vi "read_inverter (SubVI).vi"(8 "error in (no error)":errorcluster, 11 "Modbus Master in":refnum<class "Modbus Master.lvclass">) -> (0 "error out":errorcluster, 3 "Modbus Master out":refnum<class "Modbus Master.lvclass">)   [LabVIEW 2024, in "SALICRU_MODBUS.lvlib"]
uses:
  SALICRU_MODBUS.lvlib
  <vilib>/Modbus/master/Modbus Master.lvclass
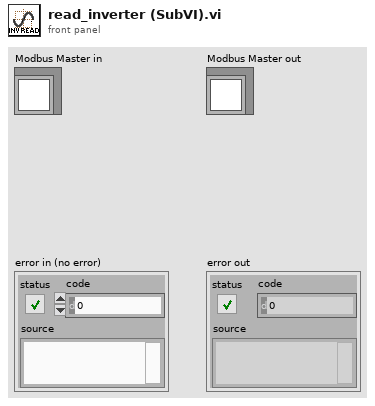
[diagram p1: front panel]
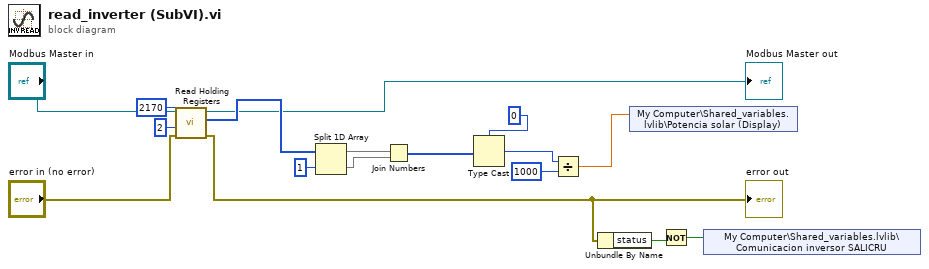
[diagram p0: block diagram]
diagram:
  n1 = call-dynamic "Read Holding Registers.vi"("error in (no error)"="error in (no error)", "number of holding registers"=u16 2, "starting address"=u16 2170, "Modbus master in"="Modbus Master in") -> ("error out"=w2:errorcluster, "register values"=w8:u16[], "Modbus master out"=→"Modbus Master out":refnum<class "Modbus Master.lvclass">)  [unwired: 5 in]
  "error out" <- w2
  n2 = Split 1D Array(array=w8, index=1) -> (first subarray=w10:u16[], second subarray=w11:u16[])
  n3 = Join Numbers(hi=w10, lo=w11) -> ((hi.lo)=w12:u32[])
  n4 = Type Cast(type=0, x=w12) -> (*(type *) &x=w16:i32)
  n5 = Divide(x=w16, y=1000) -> (x/y=w4:dbl)
  n6 = Unbundle By Name(w2) -> ("status"=w3:bool)
  n7 = shared-variable "My Computer\\Shared_variables.lvlib\\Potencia solar (Display)"(w4) -> ()  [unwired: 1 in, 1 out]
  n8 = Not(x=w3) -> (.not. x?=w1:bool)
  n9 = shared-variable "My Computer\\Shared_variables.lvlib\\Comunicacion inversor SALICRU"(w1) -> ()  [unwired: 1 in, 1 out]
